vi "MinimalCaptureExample.vi"() -> ()   [LabVIEW 2020]
uses:
  C:/Users/Public/Documents/Photometrics/TPM-LabVIEWSamples/Examples/2020/Dependencies/PVCamNET.dll
  Public/Documents/Photometrics/TPM-LabVIEWSamples/Examples/2020/Dependencies/PVCamNET.dll
  shell32.dll
panel:
  out "Current Frame 2":u32
  out "Image Data 2":u16[][](array[numeric])
  in  "Delay":u32=1
  in  "FramesToCapture":u16=1000
  out "Frame Numbes":u32[](array[numeric])
  in  "Quit":bool
  in  "Capture":bool
  out "Image Data":u16[][](array[numeric])
  out "Error":errorcluster
  out "Current Frame":u32
  out "Sensor Width":u32
  out "Sensor Height":u32
  out "Camera Name":string
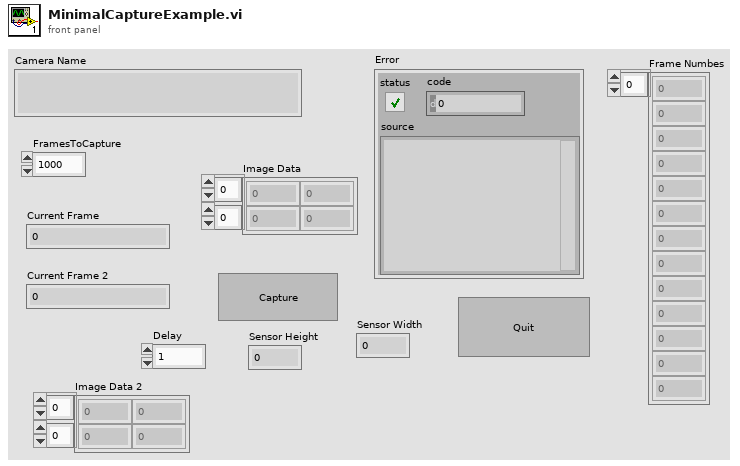
[diagram p1: front panel]
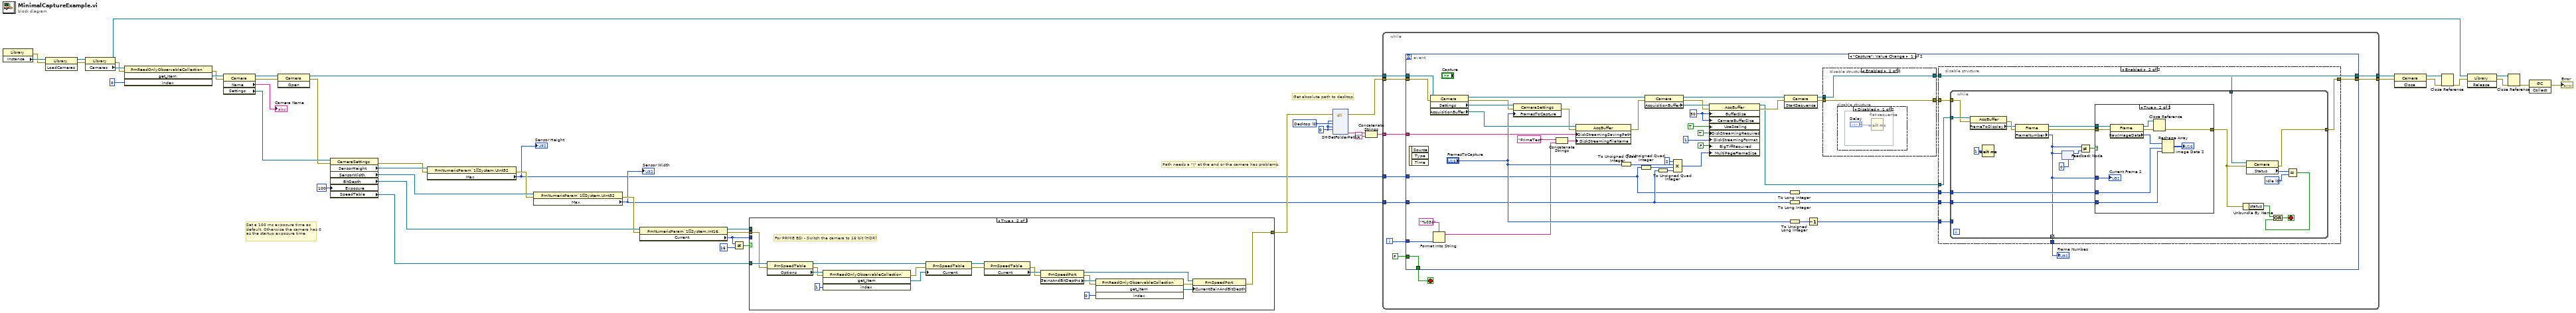
[diagram p0: block diagram]
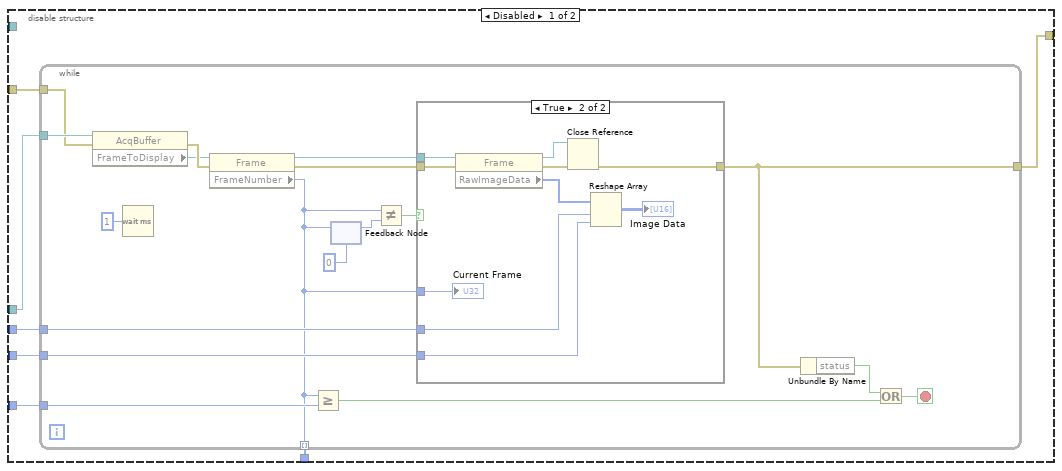
[diagram p2: hidden frame]
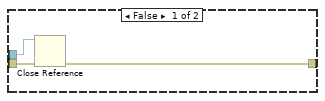
[diagram p3: hidden frame]
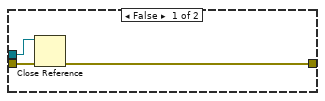
[diagram p4: hidden frame]
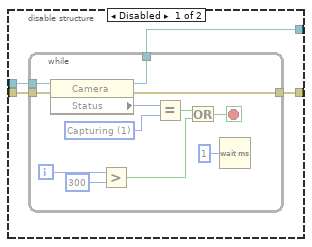
[diagram p5: hidden frame]
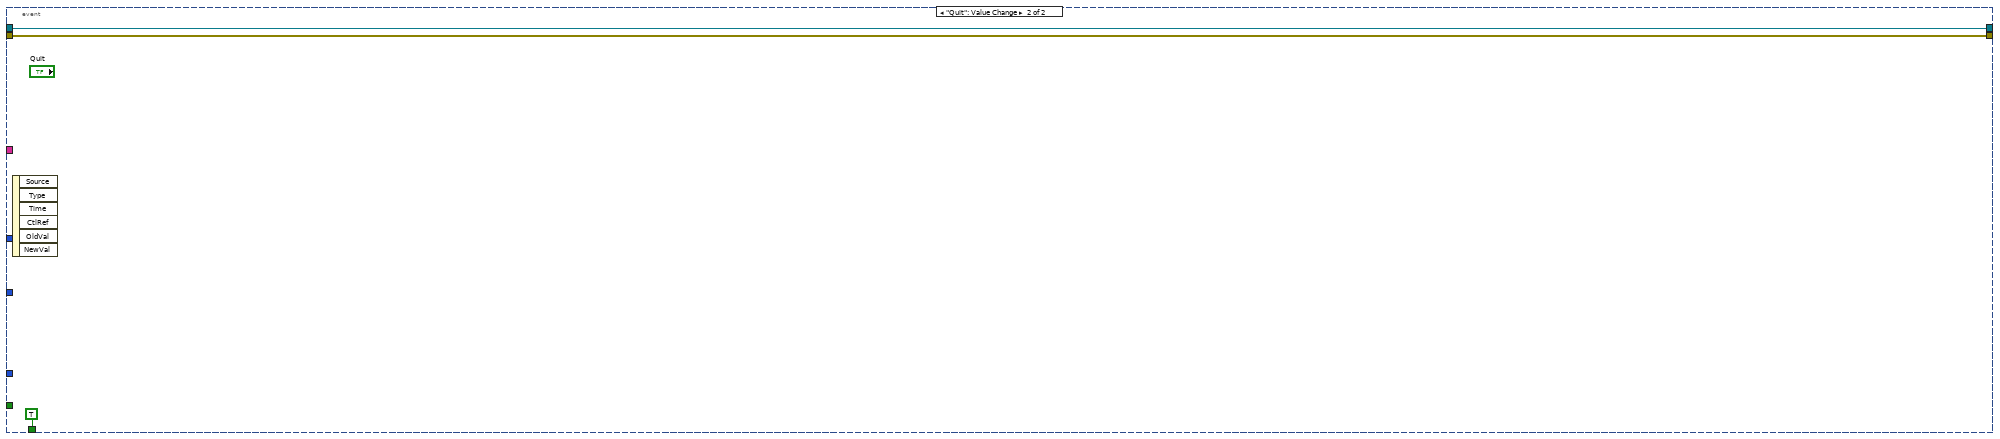
[diagram p7: hidden frame]
diagram:
  w13 = 0 items=["Desktop"=0, "Personal Documents"=5, "AppData"=26, "Local AppData"=28, "Common AppData"=35, "Program Files"=38, "Program Files Common"=43, "Common Documents"=46] ("Requested Path")
  w12 = 0 ("HWND")
  # "Path needs a \"\\\" at the end or the camera has problems."
  # "Get absolute path to desktop."
  # "Set a 100 ms exposure time as default. Otherwise the camera has 0 as the startup exposure time."
  n1 = property class="Library"() -> (error out=w44:errorcluster, "Instance"=w47:refnum<k24>)  [unwired: 2 in, 1 out]
  n2 = invoke class="Library" method="LoadCameras"(reference=w47, error in=w44) -> (reference out=w46:refnum<k24>, error out=w43:errorcluster)  [unwired: 1 in, 1 out]
  n3 = property class="Library"(reference=w46, error in=w43) -> (reference out=w32:refnum<k24>, error out=w42:errorcluster, "Cameras"=w45:refnum<k24>)
  n4 = invoke class="PmReadOnlyObservableCollection`" method="get_Item"(reference=w45, error in=w42, "index"=0) -> (error out=w40:errorcluster, "get_Item"=w41:refnum<k24>)  [unwired: 1 in, 2 out]
  n5 = property class="Camera"(reference=w41, error in=w40) -> (reference out=w38:refnum<k24>, error out=w30:errorcluster, "Name"=→"Camera Name":string, "Settings"=w39:refnum<k24>)
  n6 = invoke class="Camera" method="Open"(reference=w38, error in=w30) -> (reference out=w11:refnum<k24>, error out=w29:errorcluster)  [unwired: 1 in, 1 out]
  n7 = property class="CameraSettings"(reference=w39, error in=w29, "Exposure"=u32 100) -> (error out=w26:errorcluster, "SensorHeight"=w28:refnum<k24>, "SensorWidth"=w27:refnum<k24>, "BitDepth"=w24:refnum<k24>, "SpeedTable"=w21:refnum<k24>)  [unwired: 1 out]
  n8 = property class="PmNumericParam`1[[System.UInt32"(reference=w28, error in=w26) -> (error out=w25:errorcluster, "Max"=w1:u32)  [unwired: 1 out]
  "Sensor Height" <- w1
  n9 = property class="PmNumericParam`1[[System.UInt32"(reference=w27, error in=w25) -> (error out=w23:errorcluster, "Max"=w2:u32)  [unwired: 1 out]
  "Sensor Width" <- w2
  n10 = property class="PmNumericParam`1[[System.Int16,"(reference=w24, error in=w23) -> (reference out=w34:refnum<k24>, error out=w33:errorcluster, "Current"=w31:i16)
  n11 = Not Equal?(x=w31, y=i16 16) -> (x != y?=w35:bool)
  n12 = case shown="True" w35 {
    tunnel: w34 -> [_ _]
    tunnel: w33 -> [w48 w64]
    tunnel: [w48 w49] -> w10
    tunnel: w31 -> [_ _]
    tunnel: w21 -> [_ w67]
    frame False {
    }
    frame True {
      # "For PRMIE BSI - Switch the camera to 16 bit (HDR)"
      n13 = property class="PmSpeedTable"(reference=w67, error in=w64) -> (reference out=w62:refnum<k24>, error out=w63:errorcluster, "Options"=w66:refnum<k24>)
      n14 = invoke class="PmReadOnlyObservableCollection`" method="get_Item"(reference=w66, error in=w63, "index"=1) -> (error out=w61:errorcluster, "get_Item"=w60:refnum<k24>)  [unwired: 1 in, 2 out]
      n15 = property class="PmSpeedTable"(reference=w62, error in=w61, "Current"=w60) -> (reference out=w59:refnum<k24>, error out=w58:errorcluster)
      n16 = property class="PmSpeedTable"(reference=w59, error in=w58) -> (error out=w55:errorcluster, "Current"=w57:refnum<k24>)  [unwired: 1 out]
      n17 = property class="PmSpeedPort"(reference=w57, error in=w55) -> (reference out=w50:refnum<k24>, error out=w54:errorcluster, "GainsAndBitDepths"=w56:refnum<k24>)
      n18 = invoke class="PmReadOnlyObservableCollection`" method="get_Item"(reference=w56, error in=w54, "index"=0) -> (error out=w51:errorcluster, "get_Item"=w52:refnum<k24>)  [unwired: 1 in, 2 out]
      n19 = property class="PmSpeedPort"(reference=w50, error in=w51, "CurrentGainAndBitDepth"=w52) -> (error out=w49:errorcluster)  [unwired: 1 out]
    }
  }
  n20 = dll-call lib="shell32.dll" fn="SHGetFolderPathA"(error in=w10, "HWND"=w12, "nFolder"=w13, "hToken"=w12, "dwFlags"=w12) -> (error out=w9:errorcluster, "pszPath"=w5:string)  [unwired: 8 in, 1 out]
  n21 = Concatenate Strings(w5, "\\" ("string")) -> (w3:string)
  n22 = while {
    tunnel: w3 -> [w73]
    tunnel: w2 -> [w72]
    tunnel: w1 -> [w71]
    tunnel: w11 -> [w77]
    tunnel: [w75] -> w8
    tunnel: w9 -> [w76]
    tunnel: [w74] -> w7
    i -> [w70]
    stop <- w68 stop-if-true
    n23 = event shown="[0] \"Capture\": Value Change" {
      selector: _ -> [_ _]
      dyn-events: _ -> [_ _]
      timeout: _ -> [_ _]
      tunnel: w77 -> [w116 w223]
      tunnel: w76 -> [w115 w222]
      tunnel: [w78 w223] -> w75
      tunnel: [w95 w222] -> w74
      tunnel: w73 -> [w94 _]
      tunnel: w72 -> [w93 _]
      tunnel: w71 -> [w92 _]
      tunnel: w70 -> [w88 _]
      tunnel: [w84 TRUE] -> w68
      tunnel: FALSE -> [w84 _]
      event "Capture": Value Change {
        w103 = u32 50 ("BufferSize")
        n24 = event-data() -> ()  [unwired: 1 in, 3 out]
        n25 = property class="Camera"(reference=w116, error in=w115) -> (reference out=w102:refnum<k24>, error out=w119:errorcluster, "Settings"=w120:refnum<k24>, "AcquisitionBuffer"=w118:refnum<k24>)
        n26 = Format Into String(format string="%03d", w88) -> (resulting string=w85:string)  [unwired: 2 in, 1 out]
        n27 = property class="CameraSettings"(reference=w120, error in=w119, "FramesToCapture"="FramesToCapture") -> (error out=w117:errorcluster)  [unwired: 1 out]
        n28 = Concatenate Strings("PrimeTest", w85) -> (w86:string)
        n29 = property class="AcqBuffer"(reference=w118, error in=w117, "DiskStreamingSavingPath"=w94, "DiskStreamingFileName"=w86) -> (error out=w101:errorcluster)  [unwired: 1 out]
        n30 = To Unsigned Quad Integer(1:"FramesToCapture") -> (0:w107:u64)
        n31 = To Unsigned Quad Integer(1:w92) -> (0:w105:u64)
        n32 = property class="Camera"(reference=w102, error in=w101) -> (reference out=w100:refnum<k24>, error out=w113:errorcluster, "AcquisitionBuffer"=w114:refnum<k24>)
        n33 = To Unsigned Quad Integer(1:w93) -> (0:w106:u64)
        n34 = Compound Arithmetic op=MULTIPLY(u64 2 ("value"), w107, w105, w106) -> (w104:u64)
        n35 = property class="AcqBuffer"(reference=w114, error in=w113, "BufferSize"=w103, "CameraBufferSize"=w103, "UseScaling"=TRUE, "DiskStreamingRequired"=TRUE, "DiskStreamingFormat"=u32 1, "BigTiffRequired"=FALSE, "MultiPageFrameSize"=w104) -> (reference out=w82:refnum<k24>, error out=w99:errorcluster)
        n36 = invoke class="Camera" method="StartSequence"(reference=w100, error in=w99) -> (reference out=w81:refnum<k24>, error out=w80:errorcluster)  [unwired: 1 in, 1 out]
        n37 = To Long Integer(number=w92) -> (32bit integer=w91:i32)
        n38 = To Long Integer(number=w93) -> (32bit integer=w90:i32)
        n39 = To Unsigned Long Integer(number="FramesToCapture") -> (unsigned 32bit integer=w96:u32)
        n40 = Decrement(x=w96) -> (x-1=w98:u32)
        n41 = disable-structure shown="Enabled" {
          disable-tunnel: w81 -> [w206 w220]
          disable-tunnel: w80 -> [w205 w219]
          disable-tunnel: [w204 w220] -> w78
          disable-tunnel: [w203 w219] -> w79
          frame Disabled {
            n42 = while {
              tunnel: w206 -> [w210]
              tunnel: w205 -> [w209]
              tunnel: [w208] -> w204
              tunnel: [w207] -> w203
              i -> [w217]
              stop <- w211 stop-if-true
              w214 = 1 items=["Idle", "Capturing"] ("Status")
              n43 = property class="Camera"(reference=w210, error in=w209) -> (reference out=w208:refnum<k24>, error out=w207:errorcluster, "Status"=w215:i32)
              n44 = Greater?(x=w217, y=300) -> (0:w212:bool)
              n45 = Equal?(x=w215, y=w214) -> (x = y?=w213:bool)
              n46 = Or(x=w213, y=w212) -> (x .or. y?=w211:bool)
              n47 = Wait (ms)(milliseconds to wait=u32 1) -> ()  [unwired: 1 out]
            }
          }
          frame Enabled {
            n48 = disable-structure shown="Disabled" {
              frame Disabled {
                n49 = flat-sequence {
                  frame #0 {
                    n50 = Wait (ms)(milliseconds to wait="Delay") -> ()  [unwired: 1 out]
                  }
                }
              }
              frame Enabled {
              }
            }
          }
        }
        n51 = disable-structure shown="Enabled" {
          disable-tunnel: w98 -> [w127 w167]
          disable-tunnel: [w126 w166] -> w95
          disable-tunnel: w91 -> [w125 w165]
          disable-tunnel: w90 -> [w124 w164]
          disable-tunnel: [w123 w163] -> w83
          disable-tunnel: w82 -> [w122 w162]
          disable-tunnel: w79 -> [w121 w161]
          disable-tunnel: w78 -> [_ w160]
          frame Disabled {
            n52 = while {
              tunnel: w122 -> [w144]
              tunnel: w121 -> [w143]
              tunnel: w127 -> [w142]
              tunnel: [w130] -> w126
              tunnel: w124 -> [w132]
              tunnel: w125 -> [w133]
              tunnel: [w129] -> w123 mode=indexing
              stop <- w139 stop-if-true
              n53 = property class="AcqBuffer"(reference=w144, error in=w143) -> (error out=w146:errorcluster, "FrameToDisplay"=w145:refnum<k24>)  [unwired: 1 out]
              n54 = Wait (ms)(milliseconds to wait=u32 1) -> ()  [unwired: 1 out]
              n55 = Wait (ms)(milliseconds to wait=u32 1) -> ()  [unwired: 1 out]
              n56 = property class="Frame"(reference=w145, error in=w146) -> (reference out=w134:refnum<k24>, error out=w131:errorcluster, "FrameNumber"=w129:u32)
              n57 = Greater Or Equal?(x=w129, y=w142) -> (x >= y?=w141:bool)
              n58 = feedback #1(u32 0 ("FrameNumber")) -> (w136:u32)
              n59 = feedback-in #1(w129) -> ()
              n60 = Not Equal?(x=w129, y=w136) -> (x != y?=w135:bool)
              n61 = case shown="True" w135 {
                tunnel: w134 -> [w147 w159]
                tunnel: w133 -> [_ w158]
                tunnel: w132 -> [_ w157]
                tunnel: w131 -> [w149 w156]
                tunnel: [w148 w150] -> w130
                tunnel: w129 -> [_ w155]
                frame False {
                  n62 = Close Reference(reference=w147, error in (no error)=w149) -> (error out=w148:errorcluster)
                }
                frame True {
                  n63 = property class="Frame"(reference=w159, error in=w156) -> (reference out=w152:refnum<k24>, error out=w151:errorcluster, "RawImageData"=w153:u16[])
                  n64 = Close Reference(reference=w152, error in (no error)=w151) -> (error out=w150:errorcluster)
                  n65 = Reshape Array(w153, w158, w157) -> (→"Image Data":u16[][])
                  "Current Frame" <- w155
                }
              }
              n66 = Unbundle By Name(w130) -> ("status"=w140:bool)
              n67 = Or(x=w140, y=w141) -> (x .or. y?=w139:bool)
            }
          }
          frame Enabled {
            n68 = while {
              tunnel: w162 -> [w187]
              tunnel: w161 -> [w186]
              tunnel: w167 -> [_]
              tunnel: [w168] -> w166
              tunnel: w164 -> [w177]
              tunnel: w165 -> [w178]
              tunnel: [w175] -> w163 mode=indexing
              tunnel: w160 -> [w171]
              stop <- w184 stop-if-true
              w173 = 0 items=["Idle", "Capturing"] ("Status")
              n69 = property class="AcqBuffer"(reference=w187, error in=w186) -> (error out=w189:errorcluster, "FrameToDisplay"=w188:refnum<k24>)  [unwired: 1 out]
              n70 = Wait (ms)(milliseconds to wait=u32 1) -> ()  [unwired: 1 out]
              n71 = Wait (ms)(milliseconds to wait=u32 1) -> ()  [unwired: 1 out]
              n72 = property class="Frame"(reference=w188, error in=w189) -> (reference out=w179:refnum<k24>, error out=w176:errorcluster, "FrameNumber"=w175:u32)
              n73 = feedback #2(u32 0 ("FrameNumber")) -> (w181:u32)
              n74 = feedback-in #2(w175) -> ()
              n75 = Not Equal?(x=w175, y=w181) -> (x != y?=w180:bool)
              n76 = case shown="True" w180 {
                tunnel: w179 -> [w190 w202]
                tunnel: w178 -> [_ w201]
                tunnel: w177 -> [_ w200]
                tunnel: w176 -> [w192 w199]
                tunnel: [w191 w193] -> w169
                tunnel: w175 -> [_ w198]
                frame False {
                  n77 = Close Reference(reference=w190, error in (no error)=w192) -> (error out=w191:errorcluster)
                }
                frame True {
                  n78 = property class="Frame"(reference=w202, error in=w199) -> (reference out=w195:refnum<k24>, error out=w194:errorcluster, "RawImageData"=w196:u16[])
                  n79 = Close Reference(reference=w195, error in (no error)=w194) -> (error out=w193:errorcluster)
                  n80 = Reshape Array(w196, w201, w200) -> (→"Image Data 2":u16[][])
                  "Current Frame 2" <- w198
                }
              }
              n81 = Unbundle By Name(w169) -> ("status"=w185:bool)
              n82 = property class="Camera"(reference=w171, error in=w169) -> (error out=w168:errorcluster, "Status"=w172:i32)  [unwired: 1 out]
              n83 = Equal?(x=w172, y=w173) -> (x = y?=w170:bool)
              n84 = Or(x=w185, y=w170) -> (x .or. y?=w184:bool)
            }
          }
        }
        "Frame Numbes" <- w83
      }
      event "Quit": Value Change {
        n85 = event-data() -> ()  [unwired: 1 in, 6 out]
      }
    }
  }
  n86 = invoke class="Camera" method="Close"(reference=w8, error in=w7) -> (reference out=w18:refnum<k24>, error out=w16:errorcluster)  [unwired: 1 in, 1 out]
  n87 = Close Reference(reference=w18, error in (no error)=w16) -> (error out=w15:errorcluster)
  n88 = invoke class="Library" method="Release"(reference=w32, error in=w15) -> (reference out=w17:refnum<k24>, error out=w20:errorcluster)  [unwired: 1 in, 1 out]
  n89 = Close Reference(reference=w17, error in (no error)=w20) -> (error out=w19:errorcluster)
  n90 = invoke class="GC" method="Collect"(error in=w19) -> (error out=→"Error":errorcluster)  [unwired: 2 in, 2 out]
